vi "main - ONE Motor.vi"() -> ()   [LabVIEW 2018]
uses:
  Ctls/LoggingRate.ctl
  Ctls/MotorConfig.ctl
  Ctls/MotroConfigData.ctl
  Ctls/MagType.ctl
  Ctls/QueueData.ctl
  Ctls/State.ctl
  Ctls/CmdData.ctl
  Ctls/ConsumerLoopData.ctl
  Ctls/DisplayIndicator.ctl
  Ctls/DatabaseCmd.ctl
  <vilib>/Analysis/baseanly.llb/Mean (DBL).vi
  Siemens S7 TCP v3_3 LV 8_5/Siemens S7 TCP v3_3 LV 8_5/S7 TCP API Library/S7 TCP.lvlib
  <vilib>/Analysis/NI_AALBase.lvlib
panel:
  out "error out":errorcluster
  out "Motor#1_EmoStop?":bool caption="急停指示"
  in  "Speed Setting Checked?_4":bool
  in  "Speed Setting Checked?_3":bool
  in  "Speed Setting Checked?_2":bool
  in  "Speed Setting Checked?_1":bool
  in  "Motor_SpeedSetting#4":dbl caption="电机速度设定 1" min=0.0 max=50.0 format="%.3f"
  in  "Motor_SpeedSetting#3":dbl caption="电机速度设定 1" min=0.0 max=50.0 format="%.3f"
  in  "Motor_SpeedSetting#2":dbl caption="电机速度设定 1" min=0.0 max=50.0 format="%.3f"
  out "Motor#1_Speed":sgl(knob) caption="电机转速RPS" scale=0.01..50.0 scale format="%#.3f"
  out "Motor#1_ConfigData":T1 caption="电机配置数据"
  in  "Motor#1_Config":T2 caption="电机配置"
  in  "Motor#1_SpeedSet?":bool
  in  "Log Length":i32=100
  in  "Logging Rate":T4=enum."40Hz"
  in  "sample interval (ms)":i32
  in  "Record":bool
  out "Speed Log to Display":string[][](table)
  out "Data Read":u8[][](array[numeric])
  out "Float Data Valid?":bool[](array[boolean])
  out "Bool Data Valid":bool
  in  "Stop Button":bool
  out "SpeedCurve":sgl(graph) caption="实时显示"
  in  "ClearFault?":bool caption="故障复位"
  out "Motor#1_Fault?":bool caption="故障指示 1"
  out "Motor#1_Running?":bool caption="电机运行指示"
  out "Motor#1_Connected？":bool caption="远程允许"
  out "Motor#1_Current":dbl caption="电机电流   1" format="%1.2f"
  in  "Motor_SpeedSetting#1":dbl caption="电机速度设定 1" min=0.0 max=50.0 format="%.3f"
  in  "Motor#1_Start?":bool caption="电机启动   1"
  in  "Motor#1_Direction":bool caption="电机方向\n正转          反转    1"
  # "1#大电机"
  # "RPS"
  # "RPS"
  # "RPS"
  # "RPS"
  # "A"
  # "注意：切换励磁请手动更改驱动器参数P50082,\n 当P50082=0时为永磁，P50082=1时为励磁！！"
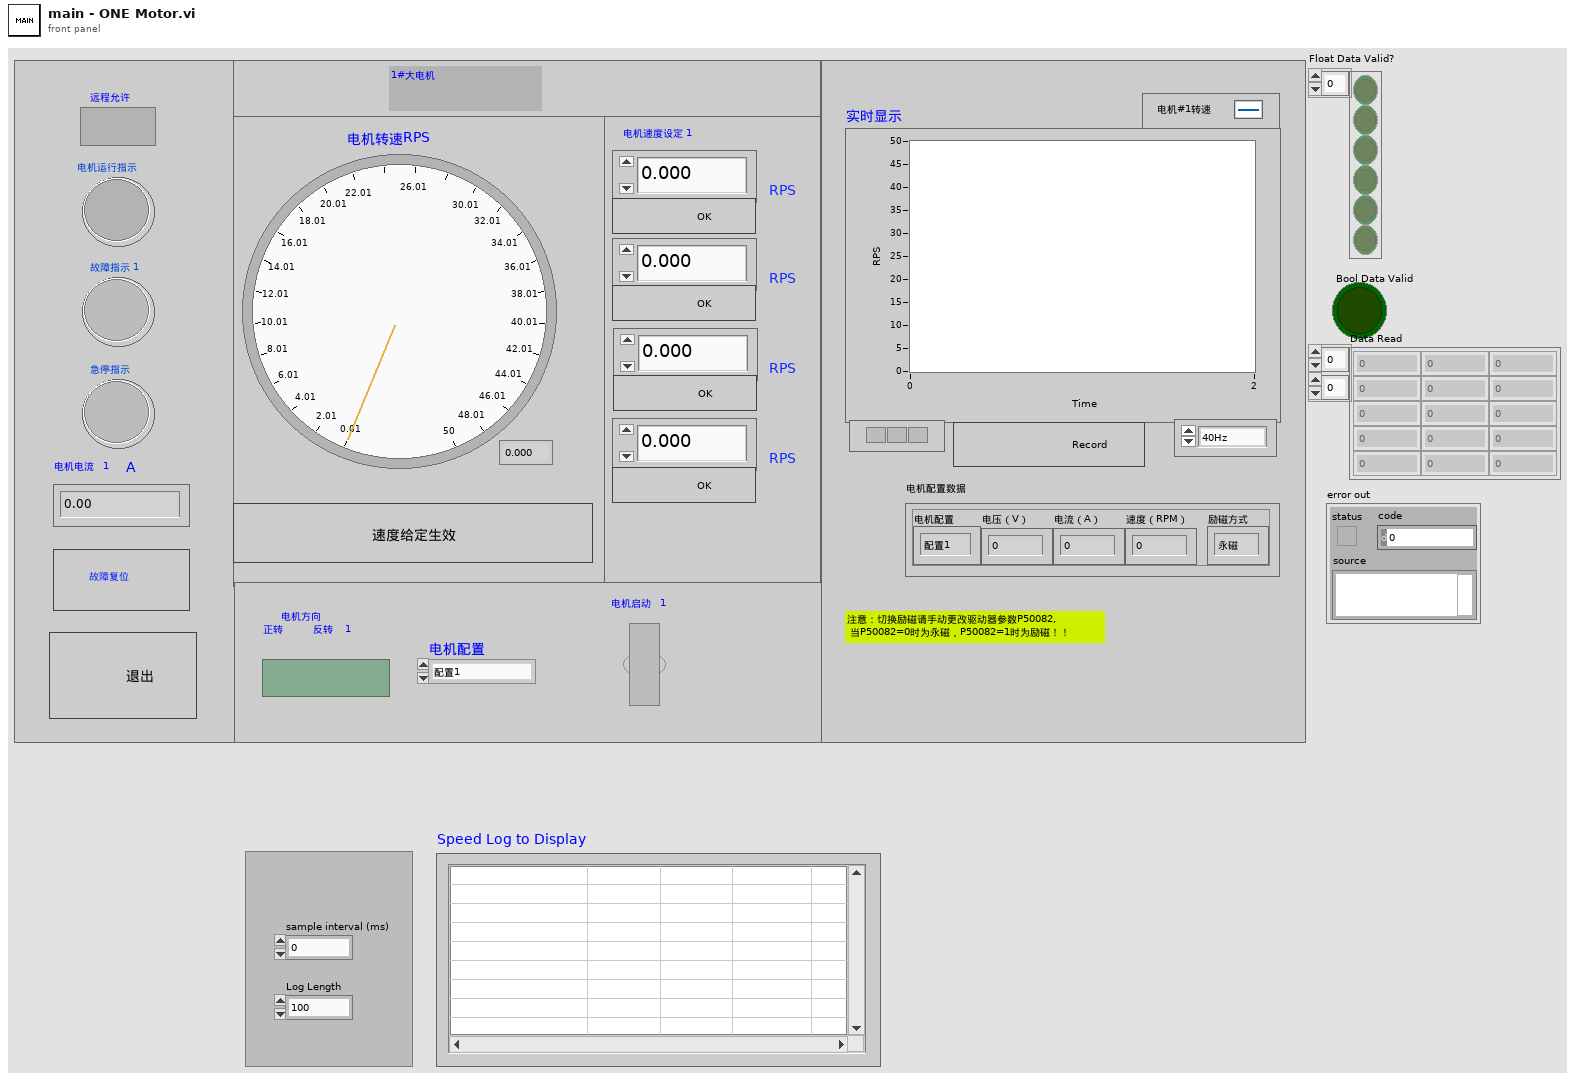
[diagram p1: front panel]
types:
  T1 = typedef "MotroConfigData.ctl" = cluster{"电机配置":T2, "电压（V）":dbl, "电流（A）":dbl, "速度（RPM）":dbl, "励磁方式":T3}
  T2 = typedef "MotorConfig.ctl" = enum16{"配置1", "配置2", "配置3", "配置4"}
  T3 = typedef "MagType.ctl" = enum16{"永磁", "励磁"}
  T4 = typedef "LoggingRate.ctl" = enum16{"1Hz", "5Hz", "10Hz", "20Hz", "25Hz", "30Hz", "35Hz", "40Hz"}
  T5 = typedef "ConsumerLoopData.ctl" = cluster{"CmdU16":u16, "Log File Path":path, "PLC Data":T6, "TCP Connection Ref":refnum<k5>, "Config File Path":path}
  T6 = typedef "DisplayIndicator.ctl" = cluster{"CommConnected_1":bool, "Run_1?":bool, "Fault_1?":bool, "CommConnected_2":bool, "Run_2?":bool, "Fault_2?":bool, "Motor Speed 2":sgl, "Motor Speed_1":sgl, "Motor Current_1":sgl, "Motor Current_2":sgl, "Motor1ConfigData":T1, "Motor2ConfigData":T1, "EmoStop_1?":bool}
  T7 = typedef "State.ctl" = enum16{"poll log data command", "poll control command", "display update", "init", "send bool command", "send float command", "datalog", "error", "fix rating rpm 1", "fix rating rpm 2", "fix both rating rpm", "fix rating rpm all", "terminate", "log Motor Speed Setting"}
  T8 = typedef "QueueData.ctl" = cluster{"State":T7, "Command Data":T9}
  T9 = typedef "CmdData.ctl" = cluster{"Address Areas":u8, "Data Block #":u16, "Start Address (bytes)":u32, "Write Data Float":sgl, "Bit #":u16, "Write Data Boolean":bool}
  T10 = typedef "DatabaseCmd.ctl" = enum16{"Insert Table Title", "Add One Record", "Delete Record", "Get Table Records", "Clear"}
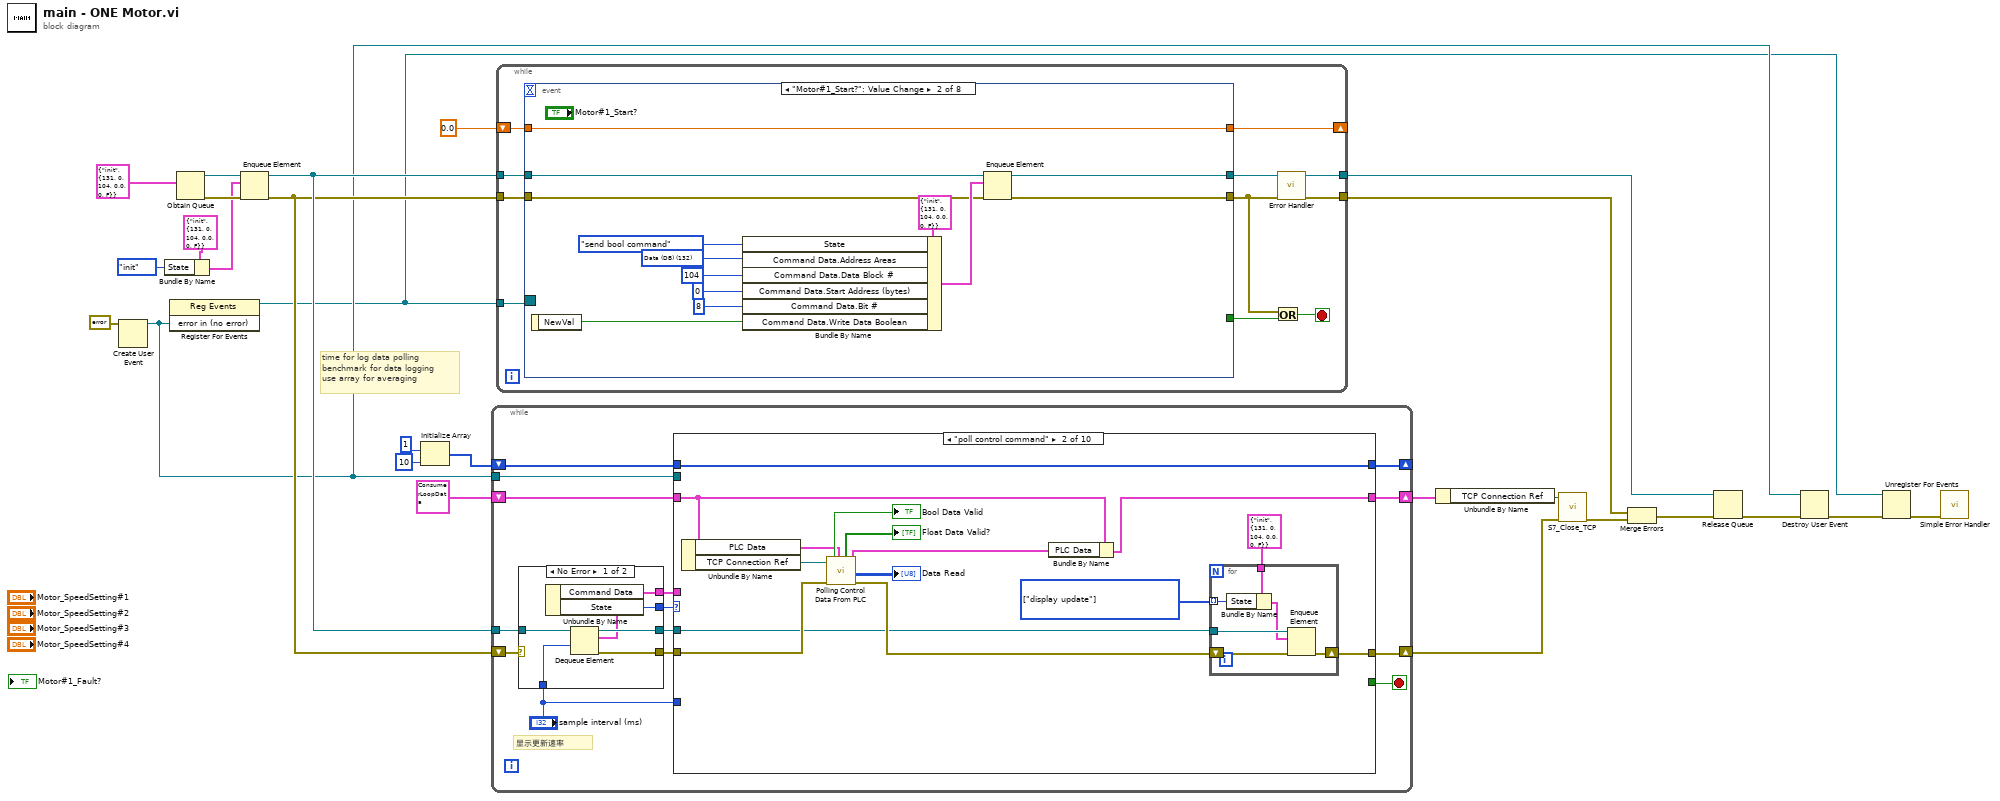
[diagram p0: block diagram]
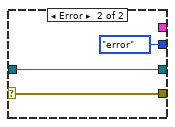
[diagram p2: hidden frame]
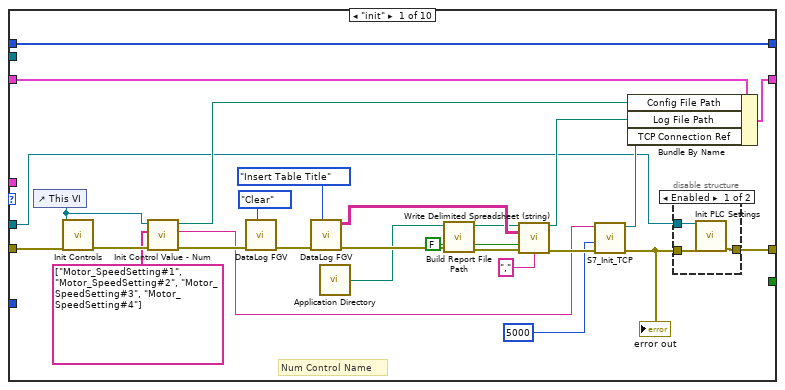
[diagram p3: hidden frame]
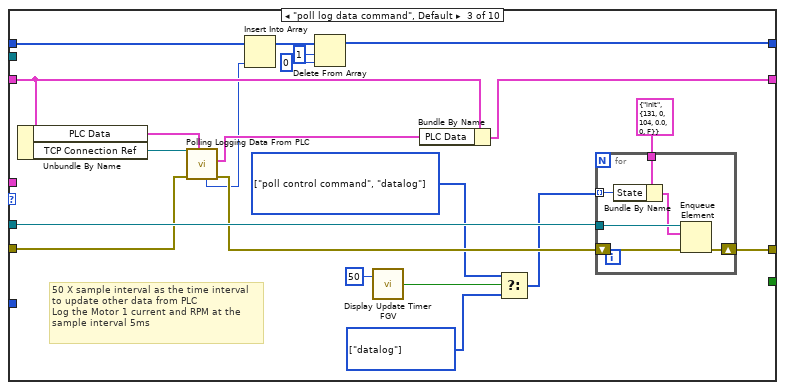
[diagram p5: hidden frame]
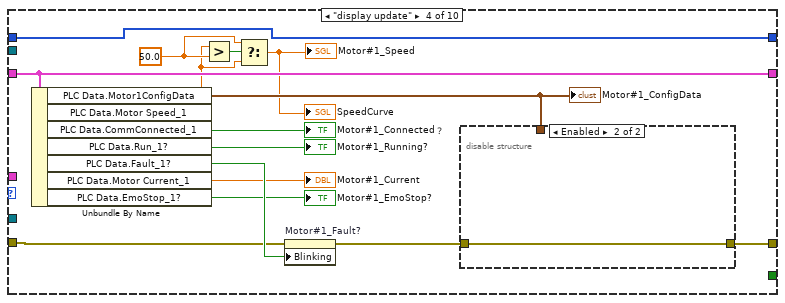
[diagram p6: hidden frame]
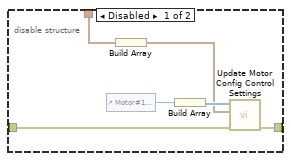
[diagram p7: hidden frame]
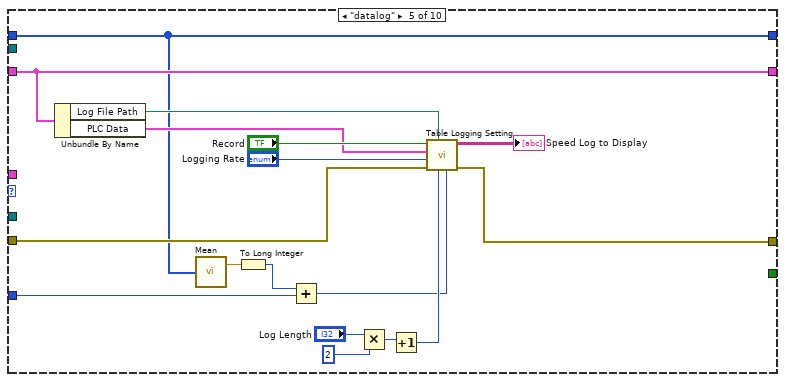
[diagram p8: hidden frame]
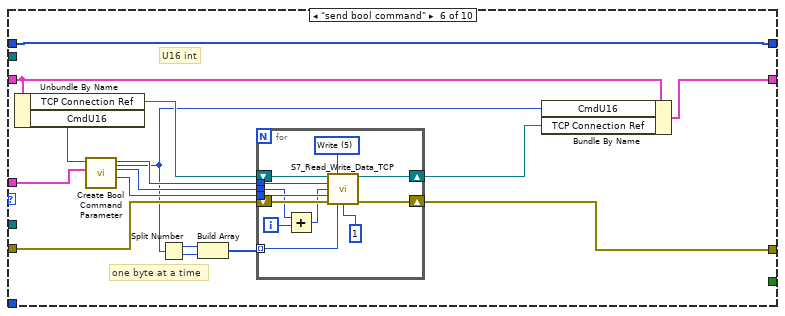
[diagram p9: hidden frame]
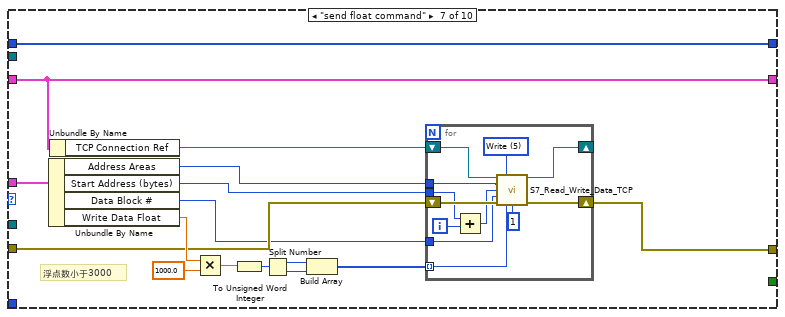
[diagram p10: hidden frame]
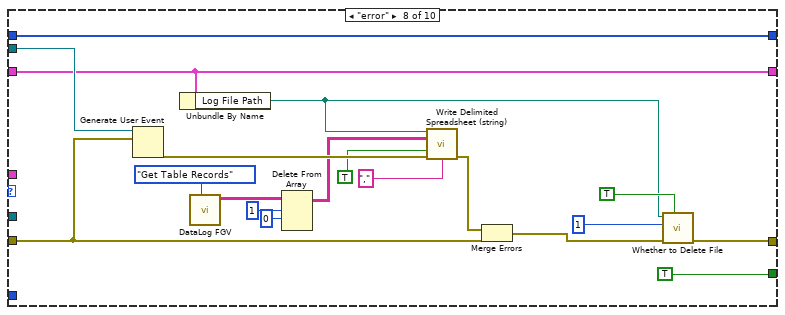
[diagram p11: hidden frame]
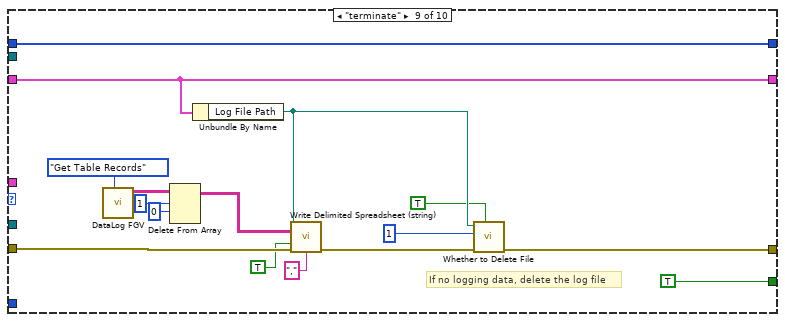
[diagram p12: hidden frame]
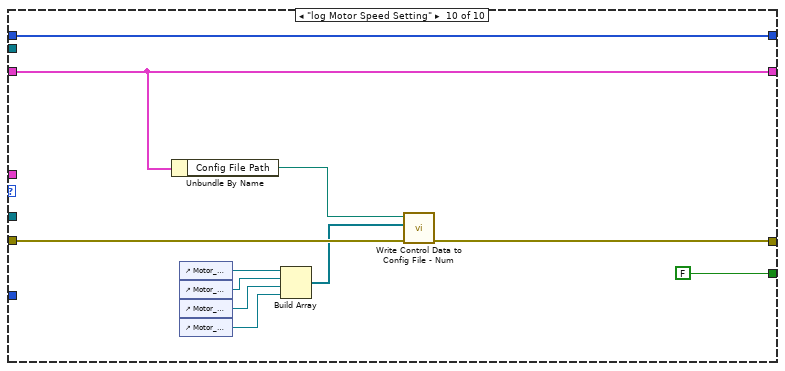
[diagram p13: hidden frame]
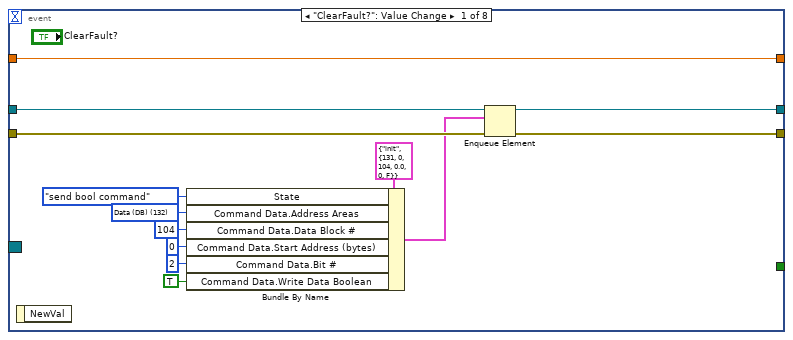
[diagram p14: hidden frame]
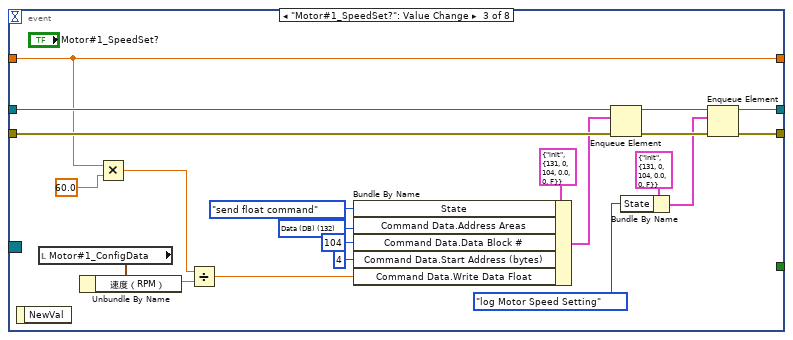
[diagram p15: hidden frame]
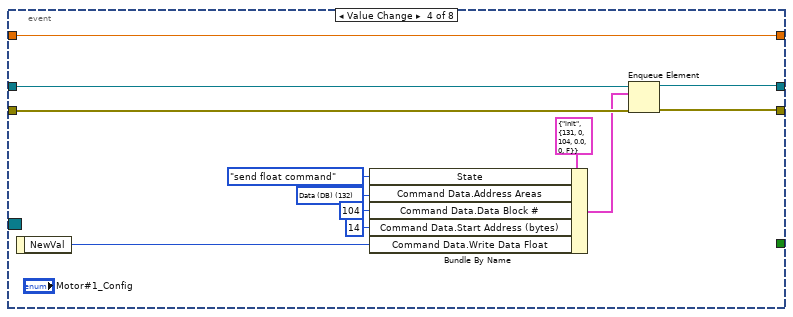
[diagram p16: hidden frame]
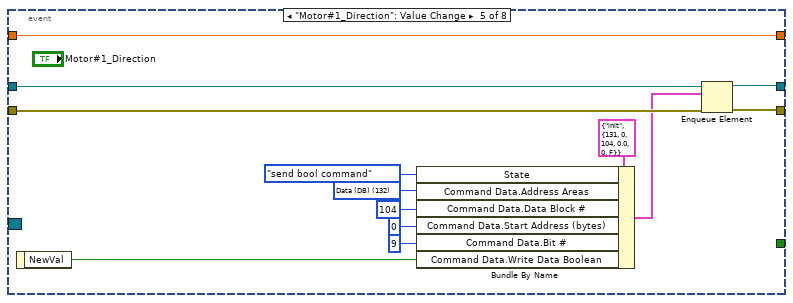
[diagram p17: hidden frame]
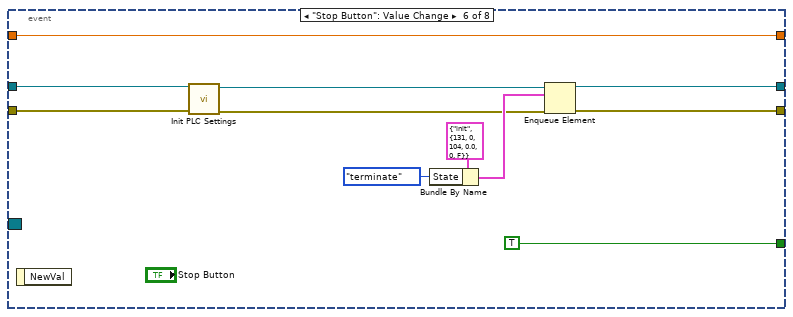
[diagram p18: hidden frame]
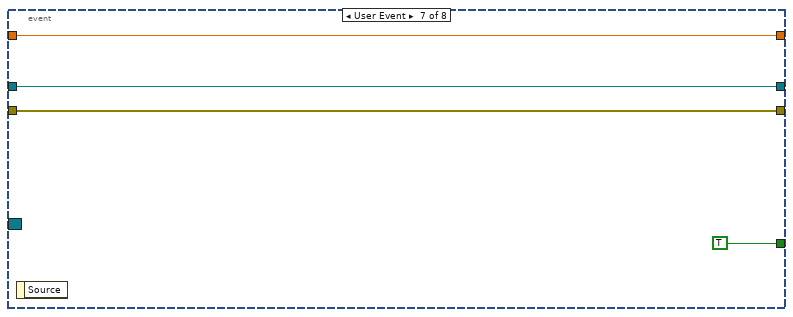
[diagram p19: hidden frame]
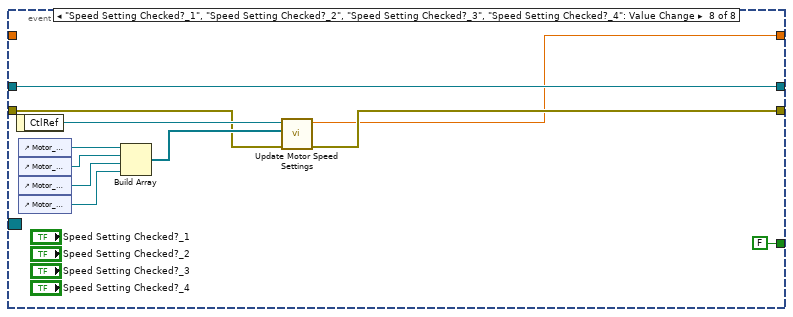
[diagram p20: hidden frame]
diagram:
  # "time for log data polling\nbenchmark for data logging\nuse array for averaging"
  n1 = Create User Event(user event datatype=errorcluster {"status"=FALSE, "code"=0, "source"=""} ("error in (no error)")) -> (user event=w17:refnum<user-event>)  [unwired: 1 in, 1 out]
  n2 = Bundle By Name(cluster=T8 {"State"=enum."init", "Command Data"={"Address Areas"=131, "Data Block #"=0, "Start Address (bytes)"=104, "Write Data Float"=0.0, "Bit #"=0, "Write Data Boolean"=FALSE}} ("element"), "State"=State."init") -> (w19:T8)
  n3 = register-events(w17) -> (reference out=w15:refnum<event-registration>)  [unwired: 2 in, 1 out]
  n4 = Obtain Queue(element data type=T8 {"State"=enum."init", "Command Data"={"Address Areas"=131, "Data Block #"=0, "Start Address (bytes)"=104, "Write Data Float"=0.0, "Bit #"=0, "Write Data Boolean"=FALSE}} ("QData")) -> (queue out=w25:refnum<queue>, error out=w23:errorcluster)  [unwired: 4 in, 1 out]
  n5 = Enqueue Element(queue=w25, element=w19, error in (no error)=w23) -> (queue out=w24:refnum<queue>, error out=w22:errorcluster)  [unwired: 1 in, 1 out]
  n6 = Initialize Array(u32 1 ("Elapsed Time(ms)"), 10 ("dimension size")) -> (w1:u32[])
  n7 = while {
    tunnel: w24 -> [w36]
    tunnel: w17 -> [w39]
    shift-right: [w37] -> w14
    shift-left: w22 -> [w38]
    shift-right: [w34] -> w12
    shift-left: T5 {"CmdU16"=0, "Log File Path"=path "", "PLC Data"={"CommConnected_1"=FALSE, "Run_1?"=FALSE, "Fault_1?"=FALSE, "CommConnected_2"=FALSE, "Run_2?"=FALSE, "Fault_2?"=FALSE, "Motor Speed 2"=0.0, "Motor Speed_1"=0.0, "Motor Current_1"=0.0, "Motor Current_2"=0.0, "Motor1ConfigData"={"电机配置"=enum."配置1", "电压（V）"=0.0, "电流（A）"=0.0, "速度（RPM）"=0.0, "励磁方式"=enum."永磁"}, "Motor2ConfigData"={"电机配置"=enum."配置1", "电压（V）"=0.0, "电流（A）"=0.0, "速度（RPM）"=0.0, "励磁方式"=enum."永磁"}, "EmoStop_1?"=FALSE}, "TCP Connection Ref"=refnum, "Config File Path"=path ""} ("Consumer Loop Data") -> [w35]
    shift-right: [w28] -> _
    shift-left: w1 -> [w27]
    stop <- w40 stop-if-true
    # "显示更新速率"
    n8 = case shown="No Error" w38 {
      selector: w38 -> [_ w50]
      tunnel: [w47 w49] -> w33
      tunnel: [w46 w50] -> w32
      tunnel: [w44 State."error" ("State")] -> w31
      tunnel: [w43 _] -> w30
      tunnel: w36 -> [w42 w49]
      tunnel: "sample interval (ms)" -> [w41 _]
      frame No Error {
        n9 = Dequeue Element(queue=w42, timeout in ms (-1)=w41) -> (queue out=w47:refnum<queue>, element=w45:T8, error out=w46:errorcluster)  [unwired: 1 in, 1 out]
        n10 = Unbundle By Name(w45) -> ("Command Data"=w43:T9, "State"=w44:T7)
      }
      frame Error {
      }
    }
    n11 = case shown="\"poll control command\"" w31 {
      tunnel: w33 -> [w53 w93 w122 _ _ _ _ _ _ _]
      tunnel: w32 -> [w63 w96 w115 w141 w166 w184 w206 w241 w254 w268]
      tunnel: [w64 w94 w123 w144 w165 w176 w200 w227 w248 w262] -> w37
      tunnel: w30 -> [_ _ _ _ _ w183 w212 _ _ _]
      tunnel: [_ _ _ _ _ _ _ TRUE ("Data Valid") TRUE ("Data Valid") FALSE ("Data Valid")] -> w40
      tunnel: w39 -> [_ _ _ _ _ _ _ w242 _ _]
      tunnel: w35 -> [w62 w90 w120 w143 w157 w173 w198 w231 w250 w270]
      tunnel: [w61 w88 w119 w143 w157 w170 w198 w231 w250 w270] -> w34
      tunnel: "sample interval (ms)" -> [_ _ _ _ w156 _ _ _ _ _]
      tunnel: [w51 w82 w103 w130 w155 w169 w197 w225 w244 w260] -> w28
      tunnel: w27 -> [w51 w82 w108 w130 w155 w169 w197 w225 w244 w260]
      frame "init" {
        # "Num Control Name"
        n12 = control-ref of="This VI"() -> (w54:refnum<vi>)
        n13 = call "Init Controls.vi"("error in"=w63, "VI ref"=w54) -> ("error out"=w60:errorcluster)  [unwired: 9 in]
        n14 = call "Init Control Value - Num.vi"("error in (no error)"=w60, "Num Control Names"=string[] ["Motor_SpeedSetting#1", "Motor_SpeedSetting#2", "Motor_SpeedSetting#3", "Motor_SpeedSetting#4"], "This VI"=w54) -> ("error out"=w59:errorcluster, "PLC IP"=w52:string, "Config File Path"=w56:path)  [unwired: 6 in]
        n15 = call "DataLog FGV.vi"("Method"=DatabaseCmd."Clear", "error in (no error)"=w59) -> ("error out"=w77:errorcluster)  [unwired: 7 in, 2 out]
        n16 = call "DataLog FGV.vi"("Method"=DatabaseCmd."Insert Table Title", "error in (no error)"=w77) -> ("error out"=w76:errorcluster, "Speed Log"=w75:string[][])  [unwired: 7 in, 1 out]
        n17 = call <vilib>:"Application Directory.vi"() -> ("Application Directory"=w69:path)
        n18 = call "Build Report File Path.vi"("error in (no error)"=w76, "File Path in"=w69) -> ("error out"=w73:errorcluster, "Report Path out"=w74:path)  [unwired: 8 in]
        n19 = call "Write Delimited Spreadsheet (string).vi"("Path"=w74, "2D data"=w75, "append to file?"=FALSE ("append to file? (new file:F)"), "error in"=w73, "delimiter (\\t)"="," ("delimiter (\\t)")) -> ("path"=w57:path, "error out"=w67:errorcluster)  [unwired: 9 in]
        n20 = call "S7_Init_TCP.vi"("error in"=w67, "Connection Timeout"=u32 5000, "IP Address"=w52) -> ("error out"=w65:errorcluster, "TCP Connection Ref"=w58:refnum<k5>)  [unwired: 2 in, 5 out]
        "error out" <- w65
        n21 = Bundle By Name(cluster=w62, "Config File Path"=w56, "Log File Path"=w57, "TCP Connection Ref"=w58) -> (w61:T5)
        n22 = disable-structure shown="Enabled" {
          disable-tunnel: w65 -> [w80 w81]
          disable-tunnel: [w79 w81] -> w64
          disable-tunnel: w53 -> [w78 _]
          frame Enabled {
            n23 = call "Init PLC Settings.vi"("error in"=w80, "queue in"=w78) -> ("error out"=w79:errorcluster)  [unwired: 8 in, 1 out]
          }
          frame Disabled {
          }
        }
      }
      frame "poll control command" {
        w91 = T7[] [enum."display update"] items=["poll log data command", "poll control command", "display update", "init", "send bool command", "send float command", "datalog", "error", "fix rating rpm 1", "fix rating rpm 2", "fix both rating rpm", "fix rating rpm all", "terminate", "log Motor Speed Setting"]
        n24 = Unbundle By Name(w90) -> ("PLC Data"=w83:T6, "TCP Connection Ref"=w87:refnum<k5>)
        n25 = call "Polling Control Data From PLC.vi"("Polling Data Input"=w83, "error in (no error)"=w96, "TCP Network Connection in"=w87) -> ("error out"=w95:errorcluster, "Data Read"=→"Data Read":u8[][], "PLC Data out"=w89:T6, "Bool Data Valid"=→"Bool Data Valid":bool, "Float Data Valid?"=→"Float Data Valid?":bool[])  [unwired: 2 in, 2 out]
        n26 = Bundle By Name(cluster=w90, "PLC Data"=w89) -> (w88:T5)
        n27 = for {
          tunnel: w93 -> [w100]
          shift-right: [w101] -> w94
          shift-left: w95 -> [w102]
          tunnel: T8 {"State"=enum."init", "Command Data"={"Address Areas"=131, "Data Block #"=0, "Start Address (bytes)"=104, "Write Data Float"=0.0, "Bit #"=0, "Write Data Boolean"=FALSE}} ("QData") -> [w98]
          tunnel: w91 -> [w97] mode=indexing
          n28 = Bundle By Name(cluster=w98, "State"=w97) -> (w99:T8)
          n29 = Enqueue Element(queue=w100, element=w99, error in (no error)=w102) -> (error out=w101:errorcluster)  [unwired: 1 in, 2 out]
        }
      }
      frame "poll log data command", Default {
        w110 = T7[] [enum."poll control command", enum."datalog"] items=["poll log data command", "poll control command", "display update", "init", "send bool command", "send float command", "datalog", "error", "fix rating rpm 1", "fix rating rpm 2", "fix both rating rpm", "fix rating rpm all", "terminate", "log Motor Speed Setting"] ("t")
        w111 = T7[] [enum."datalog"] items=["poll log data command", "poll control command", "display update", "init", "send bool command", "send float command", "datalog", "error", "fix rating rpm 1", "fix rating rpm 2", "fix both rating rpm", "fix rating rpm all", "terminate", "log Motor Speed Setting"]
        # "50 X sample interval as the time interval\nto update other data from PLC\nLog the Motor 1 current and RPM at the\nsample interval 5ms"
        n30 = Unbundle By Name(w120) -> ("PLC Data"=w117:T6, "TCP Connection Ref"=w118:refnum<k5>)
        n31 = call "Polling Logging Data From PLC.vi"("Polling Data Input"=w117, "error in (no error)"=w115, "TCP Network Connection in"=w118) -> ("error out"=w114:errorcluster, "PLC Data out"=w116:T6, "Elapsed Time(ms)"=w107:u32)  [unwired: 2 in, 4 out]
        n32 = Insert Into Array(array=w108, new element=w107) -> (w106:u32[])  [unwired: 1 in]
        n33 = Delete From Array(array=w106, length=1, index=0) -> (array with subset deleted=w103:u32[])  [unwired: 1 out]
        n34 = call "Display Update Timer FGV.vi"("Times of Sample Rate"=u32 50) -> ("Update Control Data?"=w112:bool)  [unwired: 1 in]
        n35 = Bundle By Name(cluster=w120, "PLC Data"=w116) -> (w119:T5)
        n36 = Select(t=w110, s=w112, f=w111) -> (s? t:f=w109:T7[])
        n37 = for {
          tunnel: w122 -> [w127]
          shift-right: [w128] -> w123
          shift-left: w114 -> [w129]
          tunnel: T8 {"State"=enum."init", "Command Data"={"Address Areas"=131, "Data Block #"=0, "Start Address (bytes)"=104, "Write Data Float"=0.0, "Bit #"=0, "Write Data Boolean"=FALSE}} ("QData") -> [w125]
          tunnel: w109 -> [w124] mode=indexing
          n38 = Bundle By Name(cluster=w125, "State"=w124) -> (w126:T8)
          n39 = Enqueue Element(queue=w127, element=w126, error in (no error)=w129) -> (error out=w128:errorcluster)  [unwired: 1 in, 2 out]
        }
      }
      frame "display update" {
        w134 = sgl 50.0 ("y")
        n40 = Unbundle By Name(w143) -> ("PLC Data.Motor1ConfigData"=w136:T1, "PLC Data.Motor Speed_1"=w133:sgl, "PLC Data.CommConnected_1"=→"Motor#1_Connected？":bool, "PLC Data.Run_1?"=→"Motor#1_Running?":bool, "PLC Data.Fault_1?"=w142:bool, "PLC Data.Motor Current_1"=→"Motor#1_Current":sgl, "PLC Data.EmoStop_1?"=→"Motor#1_EmoStop?":bool)
        "Motor#1_ConfigData" <- w136
        n41 = Greater?(x=w133, y=w134) -> (0:w135:bool)
        n42 = Select(t=w134, s=w135, f=w133) -> (s? t:f=→"SpeedCurve" →"Motor#1_Speed":sgl)
        n43 = property on="Motor#1_Fault?" class="Bool (strict)"(error in=w141, "Blinking"=w142) -> (error out=w137:errorcluster)  [unwired: 1 in, 1 out]
        n44 = disable-structure shown="Enabled" {
          disable-tunnel: [w150 w151] -> w144
          disable-tunnel: w137 -> [w149 w151]
          disable-tunnel: w136 -> [w146 _]
          frame Disabled {
            n45 = control-ref of="Motor#1_Config"() -> (w148:refnum<vi>)
            n46 = Build Array(w146) -> (w145:T1[])
            n47 = Build Array(w148) -> (w147:refnum<vi>[])
            n48 = call "Update Motor Config Control Settings.vi"("error in (no error)"=w149, "Motor Config Data"=w145, "Motor Config Refs"=w147) -> ("error out"=w150:errorcluster)  [unwired: 8 in]
          }
          frame Enabled {
          }
        }
      }
      frame "datalog" {
        n49 = Unbundle By Name(w157) -> ("Log File Path"=w159:path, "PLC Data"=w158:T6)
        n50 = call-poly <vilib>:"Mean.vi"("X"=w155) -> ("mean"=w153:dbl)  [unwired: 1 out]
        n51 = To Long Integer(number=w153) -> (32bit integer=w152:i32)
        n52 = Add(x=w152, y=w156) -> (x+y=w154:i32)
        n53 = Multiply(x="Log Length", y=2) -> (x*y=w161:i32)
        n54 = Increment(x=w161) -> (x+1=w160:i32)
        n55 = call "Table Logging Setting.vi"("sample interval (ms)"=w154, "Log Length"=w160, "Log File path"=w159, "error in (no error)"=w166, "Logging Rate"="Logging Rate", "Data In"=w158, "Record"="Record") -> ("error out"=w165:errorcluster, "Speed Log to Display"=→"Speed Log to Display":string[][])  [unwired: 3 in]
      }
      frame "send bool command" {
        # "one byte at a time"
        # "U16 int"
        n56 = Unbundle By Name(w173) -> ("TCP Connection Ref"=w174:refnum<k5>, "CmdU16"=w175:u16)
        n57 = call "Create Bool Command Parameter.vi"("Command Data"=w183, "Cmd U16"=w175) -> ("Data Block #"=w180:u16, "Start Address (bytes)"=w181:u32, "Address Areas"=w182:u8, "Cmd U16 out"=w172:u16)  [unwired: 6 in]
        n58 = Split Number(x=w172) -> (hi(x)=w178:u8, lo(x)=w177:u8)
        n59 = Build Array(w178, w177) -> (w179:u8[])
        n60 = for {
          tunnel: w182 -> [w192]
          tunnel: w181 -> [w186]
          tunnel: w180 -> [w191]
          shift-right: [w193] -> w171
          shift-left: w174 -> [w196]
          shift-right: [w189] -> w176
          shift-left: w184 -> [w195]
          tunnel: w179 -> [w188] mode=indexing
          i -> [w187]
          w194 = u8 5 items=["Read"=4, "Write"=5] ("Read / Write")
          n61 = Add(x=w186, y=w187) -> (x+y=w185:u32)
          n62 = call "S7_Read_Write_Data_TCP.vi"("TCP Connection Ref"=w196, "Read / Write"=w194, "Address Areas"=w192, "Start Address (bytes)"=w185, "Data Block #"=w191, "error in"=w195, "Write Data"=w188, "Length (bytes)"=u16 1) -> ("TCP Connection Ref Out"=w193:refnum<k5>, "error out"=w189:errorcluster)  [unwired: 2 in, 4 out]
        }
        n63 = Bundle By Name(cluster=w173, "CmdU16"=w172, "TCP Connection Ref"=w171) -> (w170:T5)
      }
      frame "send float command" {
        # "浮点数小于3000"
        n64 = Unbundle By Name(w212) -> ("Address Areas"=w205:u8, "Start Address (bytes)"=w204:u32, "Data Block #"=w203:u16, "Write Data Float"=w211:sgl)
        n65 = Unbundle By Name(w198) -> ("TCP Connection Ref"=w199:refnum<k5>)
        n66 = Multiply(x=w211, y=sgl 1000.0) -> (x*y=w209:sgl)
        n67 = To Unsigned Word Integer(number=w209) -> (unsigned 16bit integer=w208:u16)
        n68 = Split Number(x=w208) -> (hi(x)=w202:u8, lo(x)=w201:u8)
        n69 = Build Array(w202, w201) -> (w207:u8[])
        n70 = for {
          shift-right: [w221] -> _
          shift-left: w199 -> [w224]
          shift-right: [w219] -> w200
          shift-left: w206 -> [w223]
          tunnel: w207 -> [w216] mode=indexing
          tunnel: w205 -> [w215]
          tunnel: w204 -> [w214]
          tunnel: w203 -> [w213]
          i -> [w218]
          w222 = u8 5 items=["Read"=4, "Write"=5] ("Read / Write")
          n71 = Add(x=w214, y=w218) -> (x+y=w217:u32)
          n72 = call "S7_Read_Write_Data_TCP.vi"("TCP Connection Ref"=w224, "Read / Write"=w222, "Address Areas"=w215, "Start Address (bytes)"=w217, "Data Block #"=w213, "error in"=w223, "Write Data"=w216, "Length (bytes)"=u16 1) -> ("TCP Connection Ref Out"=w221:refnum<k5>, "error out"=w219:errorcluster)  [unwired: 2 in, 4 out]
        }
      }
      frame "error" {
        n73 = Generate User Event(user event=w242, event data cluster=w241) -> (error out=w240:errorcluster)  [unwired: 2 in, 1 out]
        n74 = Unbundle By Name(w231) -> ("Log File Path"=w226:path)
        n75 = call "DataLog FGV.vi"("Method"=DatabaseCmd."Get Table Records") -> ("Speed Log"=w236:string[][])  [unwired: 8 in, 2 out]
        n76 = Delete From Array(array=w236, length=1, index (row)=0) -> (array with subset deleted=w233:string[][])  [unwired: 1 in, 1 out]
        n77 = call "Write Delimited Spreadsheet (string).vi"("Path"=w226, "2D data"=w233, "append to file?"=TRUE ("append to file? (new file:F)"), "error in"=w240, "delimiter (\\t)"="," ("delimiter (\\t)")) -> ("error out"=w239:errorcluster)  [unwired: 9 in, 1 out]
        n78 = Merge Errors(w239, w241) -> (w228:errorcluster)
        n79 = call "Whether to Delete File.vi"("Del Log file?"=TRUE, "error in (no error)"=w228, "Number of lines"=1, "File path"=w226) -> ("error out"=w227:errorcluster)  [unwired: 7 in]
      }
      frame "terminate" {
        # "If no logging data, delete the log file"
        n80 = call "DataLog FGV.vi"("Method"=DatabaseCmd."Get Table Records") -> ("Speed Log"=w257:string[][])  [unwired: 8 in, 2 out]
        n81 = Delete From Array(array=w257, length=1, index (row)=0) -> (array with subset deleted=w253:string[][])  [unwired: 1 in, 1 out]
        n82 = Unbundle By Name(w250) -> ("Log File Path"=w247:path)
        n83 = call "Write Delimited Spreadsheet (string).vi"("Path"=w247, "2D data"=w253, "append to file?"=TRUE ("append to file? (new file:F)"), "error in"=w254, "delimiter (\\t)"="," ("delimiter (\\t)")) -> ("error out"=w249:errorcluster)  [unwired: 9 in, 1 out]
        n84 = call "Whether to Delete File.vi"("Del Log file?"=TRUE, "error in (no error)"=w249, "Number of lines"=1, "File path"=w247) -> ("error out"=w248:errorcluster)  [unwired: 7 in]
      }
      frame "log Motor Speed Setting" {
        n85 = Unbundle By Name(w270) -> ("Config File Path"=w269:path)
        n86 = control-ref of="Motor_SpeedSetting#1"() -> (w267:refnum<vi>)
        n87 = control-ref of="Motor_SpeedSetting#2"() -> (w266:refnum<vi>)
        n88 = control-ref of="Motor_SpeedSetting#3"() -> (w265:refnum<vi>)
        n89 = control-ref of="Motor_SpeedSetting#4"() -> (w264:refnum<vi>)
        n90 = Build Array(w267, w266, w265, w264) -> (w263:refnum<vi>[])
        n91 = call "Write Control Data to Config File - Num.vi"("error in (no error)"=w268, "Num Controls"=w263, "Config File Path"=w269) -> ("error out"=w262:errorcluster)  [unwired: 8 in]
      }
    }
  }
  n92 = while {
    tunnel: w24 -> [w281]
    tunnel: w22 -> [w280]
    tunnel: w15 -> [w279]
    tunnel: [w274] -> w9
    tunnel: [w273] -> w8
    shift-right: [w272] -> _
    shift-left: 0.0 ("Motor Speed") -> [w271]
    stop <- w277 stop-if-true
    n93 = event shown="[1] \"Motor#1_Start?\": Value Change" {
      selector: w279 -> [_ _ _ _ _ _ _ _]
      dyn-events: _ -> [_ _ _ _ _ _ _ _]
      timeout: _ -> [_ _ _ _ _ _ _ _]
      tunnel: [_ _ _ _ _ TRUE ("Stop Button") TRUE ("Stop Button") FALSE ("Stop Button")] -> w278
      tunnel: w281 -> [w294 w304 w327 w339 w352 w358 w368 w373]
      tunnel: w280 -> [w293 w303 w326 w337 w350 w356 w367 w372]
      tunnel: [w289 w296 w314 w338 w351 w363 w368 w373] -> w276
      tunnel: [w290 w295 w309 w336 w349 w362 w367 w371] -> w275
      tunnel: [w282 w297 w308 w329 w341 w354 w365 w369] -> w272
      tunnel: w271 -> [w282 w297 w308 w329 w341 w354 w365 _]
      event "ClearFault?": Value Change {
        w287 = u8 132 items=["I/O (P)"=128, "Input (I)"=129, "Output (Q)"=130, "Bit Memory (M)"=131, "Data (DB)"=132, "Instance Data (DI)"=133, "Local Data (L)"=134, "Predecessor Local Data (VL)"=135] ("Address Areas")
        n94 = event-data() -> ()  [unwired: 1 in, 1 out]
        n95 = Bundle By Name(cluster=T8 {"State"=enum."init", "Command Data"={"Address Areas"=131, "Data Block #"=0, "Start Address (bytes)"=104, "Write Data Float"=0.0, "Bit #"=0, "Write Data Boolean"=FALSE}} ("QData"), "State"=State."send bool command", "Command Data.Address Areas"=w287, "Command Data.Data Block #"=u16 104 ("Data Block #"), "Command Data.Start Address (bytes)"=u32 0 ("Start Address (bytes)"), "Command Data.Bit #"=u16 2 ("Bit #"), "Command Data.Write Data Boolean"=TRUE ("Write Data Boolean")) -> (w292:T8)
        n96 = Enqueue Element(queue=w294, element=w292, error in (no error)=w293) -> (queue out=w289:refnum<queue>, error out=w290:errorcluster)  [unwired: 1 in, 1 out]
      }
      event "Motor#1_Start?": Value Change {
        w302 = u8 132 items=["I/O (P)"=128, "Input (I)"=129, "Output (Q)"=130, "Bit Memory (M)"=131, "Data (DB)"=132, "Instance Data (DI)"=133, "Local Data (L)"=134, "Predecessor Local Data (VL)"=135] ("Address Areas")
        n97 = event-data() -> ("NewVal"=w298:bool)  [unwired: 1 in]
        n98 = Bundle By Name(cluster=T8 {"State"=enum."init", "Command Data"={"Address Areas"=131, "Data Block #"=0, "Start Address (bytes)"=104, "Write Data Float"=0.0, "Bit #"=0, "Write Data Boolean"=FALSE}} ("QData"), "State"=State."send bool command", "Command Data.Address Areas"=w302, "Command Data.Data Block #"=u16 104 ("Data Block #"), "Command Data.Start Address (bytes)"=u32 0 ("Start Address (bytes)"), "Command Data.Bit #"=u16 8 ("Bit #"), "Command Data.Write Data Boolean"=w298) -> (w306:T8)
        n99 = Enqueue Element(queue=w304, element=w306, error in (no error)=w303) -> (queue out=w296:refnum<queue>, error out=w295:errorcluster)  [unwired: 1 in, 1 out]
      }
      event "Motor#1_SpeedSet?": Value Change {
        w319 = u8 132 items=["I/O (P)"=128, "Input (I)"=129, "Output (Q)"=130, "Bit Memory (M)"=131, "Data (DB)"=132, "Instance Data (DI)"=133, "Local Data (L)"=134, "Predecessor Local Data (VL)"=135] ("Address Areas")
        n100 = event-data() -> ()  [unwired: 1 in, 1 out]
        n101 = local read "Motor#1_ConfigData"() -> (w321:T1)
        n102 = Unbundle By Name(w321) -> ("速度（RPM）"=w320:dbl)
        n103 = Multiply(x=w308, y=60.0) -> (x*y=w322:dbl)
        n104 = Divide(x=w322, y=w320) -> (x/y=w316:dbl)
        n105 = Bundle By Name(cluster=T8 {"State"=enum."init", "Command Data"={"Address Areas"=131, "Data Block #"=0, "Start Address (bytes)"=104, "Write Data Float"=0.0, "Bit #"=0, "Write Data Boolean"=FALSE}} ("QData"), "State"=State."send float command", "Command Data.Address Areas"=w319, "Command Data.Data Block #"=u16 104 ("Data Block #"), "Command Data.Start Address (bytes)"=u32 4 ("Start Address (bytes)"), "Command Data.Write Data Float"=w316) -> (w325:T8)
        n106 = Enqueue Element(queue=w327, element=w325, error in (no error)=w326) -> (queue out=w315:refnum<queue>, error out=w313:errorcluster)  [unwired: 1 in, 1 out]
        n107 = Bundle By Name(cluster=T8 {"State"=enum."init", "Command Data"={"Address Areas"=131, "Data Block #"=0, "Start Address (bytes)"=104, "Write Data Float"=0.0, "Bit #"=0, "Write Data Boolean"=FALSE}} ("QData"), "State"=State."log Motor Speed Setting") -> (w310:T8)
        n108 = Enqueue Element(queue=w315, element=w310, error in (no error)=w313) -> (queue out=w314:refnum<queue>, error out=w309:errorcluster)  [unwired: 1 in, 1 out]
      }
      event Value Change {
        w333 = u8 132 items=["I/O (P)"=128, "Input (I)"=129, "Output (Q)"=130, "Bit Memory (M)"=131, "Data (DB)"=132, "Instance Data (DI)"=133, "Local Data (L)"=134, "Predecessor Local Data (VL)"=135] ("Address Areas")
        n109 = event-data() -> ("NewVal"=w330:T2)  [unwired: 1 in]
        n110 = Bundle By Name(cluster=T8 {"State"=enum."init", "Command Data"={"Address Areas"=131, "Data Block #"=0, "Start Address (bytes)"=104, "Write Data Float"=0.0, "Bit #"=0, "Write Data Boolean"=FALSE}} ("QData"), "State"=State."send float command", "Command Data.Address Areas"=w333, "Command Data.Data Block #"=u16 104 ("Data Block #"), "Command Data.Start Address (bytes)"=u32 14 ("Start Address (bytes)"), "Command Data.Write Data Float"=w330) -> (w335:T8)
        n111 = Enqueue Element(queue=w339, element=w335, error in (no error)=w337) -> (queue out=w338:refnum<queue>, error out=w336:errorcluster)  [unwired: 1 in, 1 out]
      }
      event "Motor#1_Direction": Value Change {
        w346 = u8 132 items=["I/O (P)"=128, "Input (I)"=129, "Output (Q)"=130, "Bit Memory (M)"=131, "Data (DB)"=132, "Instance Data (DI)"=133, "Local Data (L)"=134, "Predecessor Local Data (VL)"=135] ("Address Areas")
        n112 = event-data() -> ("NewVal"=w342:bool)  [unwired: 1 in]
        n113 = Bundle By Name(cluster=T8 {"State"=enum."init", "Command Data"={"Address Areas"=131, "Data Block #"=0, "Start Address (bytes)"=104, "Write Data Float"=0.0, "Bit #"=0, "Write Data Boolean"=FALSE}} ("QData"), "State"=State."send bool command", "Command Data.Address Areas"=w346, "Command Data.Data Block #"=u16 104 ("Data Block #"), "Command Data.Start Address (bytes)"=u32 0 ("Start Address (bytes)"), "Command Data.Bit #"=u16 9 ("Bit #"), "Command Data.Write Data Boolean"=w342) -> (w348:T8)
        n114 = Enqueue Element(queue=w352, element=w348, error in (no error)=w350) -> (queue out=w351:refnum<queue>, error out=w349:errorcluster)  [unwired: 1 in, 1 out]
      }
      event "Stop Button": Value Change {
        n115 = event-data() -> ()  [unwired: 1 in, 1 out]
        n116 = call "Init PLC Settings.vi"("error in"=w356, "queue in"=w358) -> ("error out"=w355:errorcluster, "queue out"=w357:refnum<queue>)  [unwired: 8 in]
        n117 = Bundle By Name(cluster=T8 {"State"=enum."init", "Command Data"={"Address Areas"=131, "Data Block #"=0, "Start Address (bytes)"=104, "Write Data Float"=0.0, "Bit #"=0, "Write Data Boolean"=FALSE}} ("QData"), "State"=State."terminate") -> (w360:T8)
        n118 = Enqueue Element(queue=w357, element=w360, error in (no error)=w355) -> (queue out=w363:refnum<queue>, error out=w362:errorcluster)  [unwired: 1 in, 1 out]
      }
      event User Event {
        n119 = event-data() -> ()  [unwired: 1 in, 1 out]
      }
      event "Speed Setting Checked?_1", "Speed Setting Checked?_2", "Speed Setting Checked?_3", "Speed Setting Checked?_4": Value Change {
        n120 = event-data() -> ("CtlRef"=w375:refnum<vi>)  [unwired: 1 in]
        n121 = control-ref of="Motor_SpeedSetting#1"() -> (w379:refnum<vi>)
        n122 = control-ref of="Motor_SpeedSetting#2"() -> (w378:refnum<vi>)
        n123 = control-ref of="Motor_SpeedSetting#3"() -> (w377:refnum<vi>)
        n124 = control-ref of="Motor_SpeedSetting#4"() -> (w376:refnum<vi>)
        n125 = Build Array(w379, w378, w377, w376) -> (w374:refnum<vi>[])
        n126 = call "Update Motor Speed Settings.vi"("error in (no error)"=w372, "Motor_Speed Setting Ref Array"=w374, "Bool RefIn"=w375) -> ("error out"=w371:errorcluster, "Motor Speed"=w369:dbl)  [unwired: 7 in]
      }
    }
    n127 = Or(x=w275, y=w278) -> (x .or. y?=w277:bool)
    n128 = call "Error Handler.vi"("error in (no error)"=w275, "queue in"=w276) -> ("error out"=w274:errorcluster, "queue out"=w273:refnum<queue>)  [unwired: 8 in]
  }
  n129 = Unbundle By Name(w12) -> ("TCP Connection Ref"=w11:refnum<k5>)
  n130 = call "S7_Close_TCP.vi"("error in"=w14, "TCP Connection Ref"=w11) -> ("error out"=w10:errorcluster)  [unwired: 1 in, 8 out]
  n131 = Merge Errors(w9, w10) -> (w7:errorcluster)
  n132 = Release Queue(queue=w8, error in (no error)=w7) -> (error out=w6:errorcluster)  [unwired: 1 in, 2 out]
  n133 = Destroy User Event(user event=w17, error in=w6) -> (error out=w16:errorcluster)
  n134 = Unregister For Events(event registration refnum=w15, error in=w16) -> (error out=w5:errorcluster)
  n135 = call <vilib>:"Simple Error Handler.vi"("error in (no error)"=w5) -> ()  [unwired: 4 in, 5 out]
